vi "Init_MessageBox.vi"(4 "Image path":path, 6 "Allow to close? (T)":bool=TRUE, 7 "MessageBox in":refnum<class "MessageBox.lvclass">, 8 "error in (no error)":errorcluster, 9 "Timeout (-1)":i32=-1, 10 "Message":string, 11 "MsgBox Title":string) -> (0 "error out":errorcluster, 3 "MessageBox out":refnum<class "MessageBox.lvclass">)   [LabVIEW 2012, in "MessageBox.lvlib" / "MessageBox.lvclass"]
doc: "Instantiates an object of class \"Message Box\"."
uses:
  MessageBox.lvclass
  MessageBox.lvclass/MessageBox.ctl
  Dialog/Dialog/Dialog.lvclass
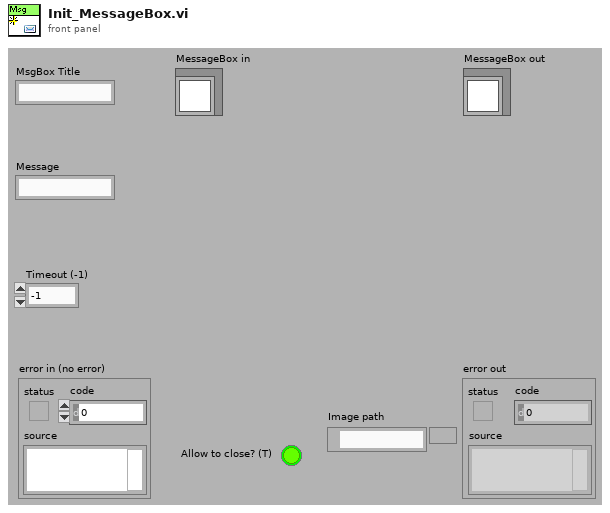
[diagram p1: front panel]
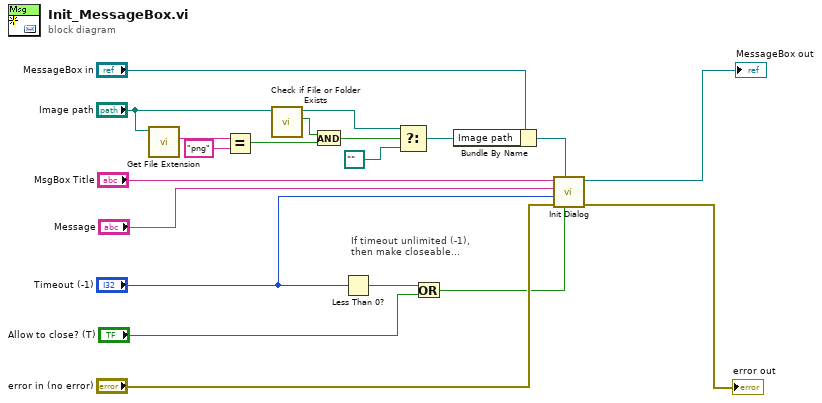
[diagram p0: block diagram]
diagram:
  # "If timeout unlimited (-1), \nthen make closeable..."
  n1 = call <vilib>:"Get File Extension.vi"("file"="Image path") -> ("lowercase file extension"=w11:string)  [unwired: 1 in, 9 out]
  n2 = Equal?(x=w11, y="png") -> (x = y?=w7:bool)
  n3 = call <vilib>:"Check if File or Folder Exists.vi"("path"="Image path") -> ("file or folder exists?"=w8:bool, "dup path"=w5:path)  [unwired: 1 in, 8 out]
  n4 = And(x=w8, y=w7) -> (x .and. y?=w6:bool)
  n5 = Less Than 0?(x="Timeout (-1)") -> (x < 0?=w17:bool)
  n6 = Select(t=w5, s=w6, f=path "") -> (s? t:f=w4:path)
  n7 = Or(x=w17, y="Allow to close? (T)") -> (x .or. y?=w15:bool)
  n8 = Bundle By Name(cluster="MessageBox in", "Image path"=w4) -> (w12:refnum<class "MessageBox.lvclass">)
  n9 = call "Init Dialog.vi"("Allow to close? (T)"=w15, "Dialog in"=w12, "error in (no error)"="error in (no error)", "Timeout (-1)"="Timeout (-1)", "Message"="Message", "Dialog Title"="MsgBox Title") -> ("error out"=→"error out":errorcluster, "Dialog out"=→"MessageBox out":refnum<class "MessageBox.lvclass">)  [unwired: 4 out]
